vi "FDTI_DX22_read_write.vi"(0 "Handle":u64, 1 "Bytes to wait for":i32, 2 "Read Answer?":bool, 3 "Bytes wait timeout / ms":i32, 5 "Clear  RxTx Buffer?":bool, 7 "Write string":string, 11 "error in (no error)":errorcluster) -> (4 "Handle out":u64, 8 "Read Data":string, 15 "error out":errorcluster)   [LabVIEW 2019]
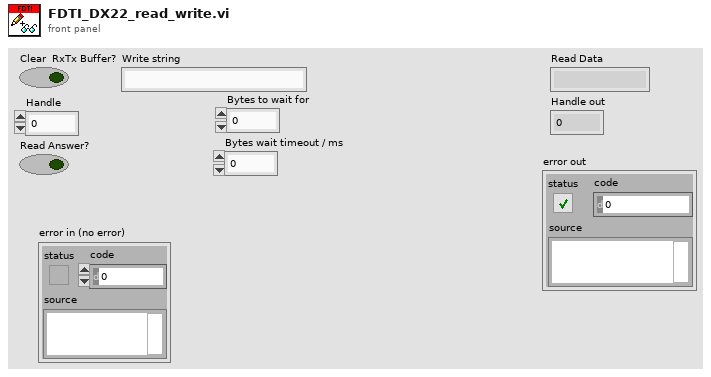
[diagram p1: front panel]
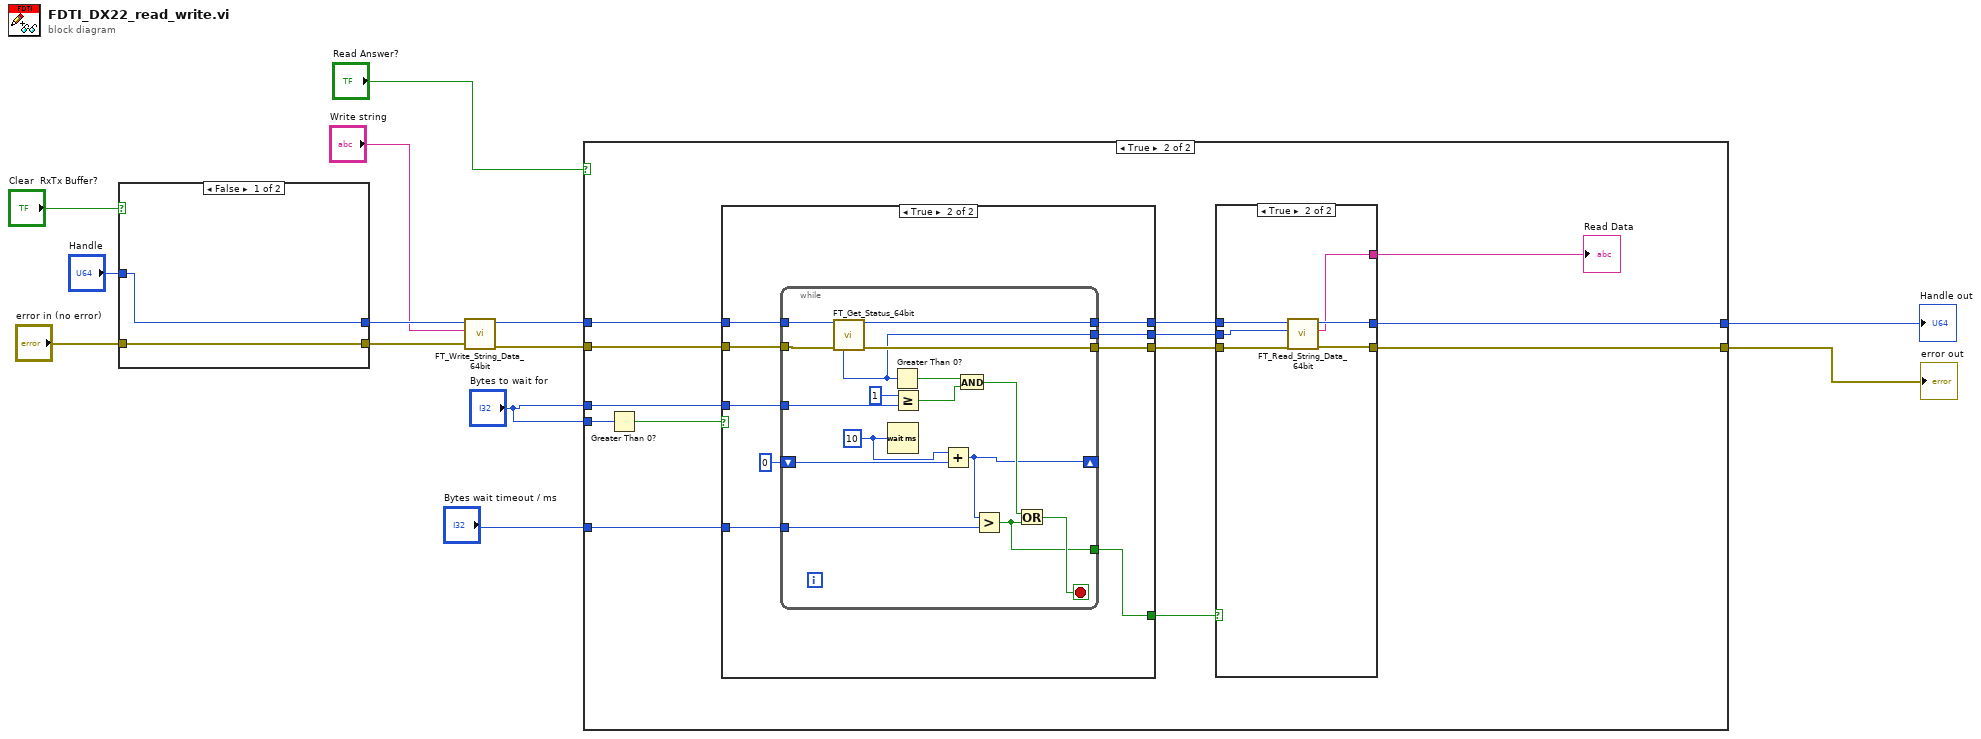
[diagram p0: block diagram]
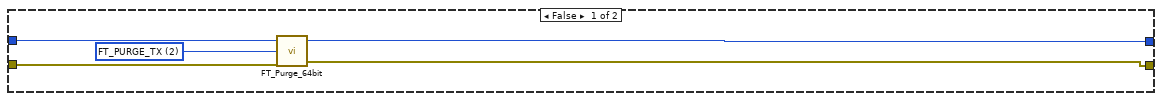
[diagram p2: hidden frame]
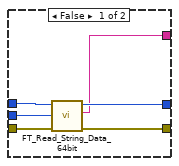
[diagram p3: hidden frame]
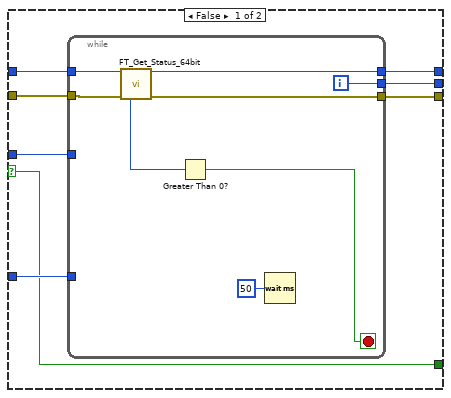
[diagram p4: hidden frame]
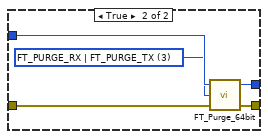
[diagram p5: hidden frame]
diagram:
  n1 = case shown="False" "Clear  RxTx Buffer?" {
    tunnel: "Handle" -> [w15 w20]
    tunnel: [w15 w19] -> w10
    tunnel: "error in (no error)" -> [w14 w17]
    tunnel: [w14 w16] -> w9
    frame False {
    }
    frame True {
      w18 = u32 3 items=["FT_PURGE_RX"=1, "FT_PURGE_TX"=2, "FT_PURGE_RX | FT_PURGE_TX"=3] ("Purge Flags")
      n2 = call "FT_Purge_64bit.vi"("error in (no error)"=w17, "Purge Flags"=w18, "Handle in"=w20) -> ("error out"=w16:errorcluster, "Handle Out"=w19:u64)  [unwired: 1 out]
    }
  }
  n3 = call "FT_Write_String_Data_64bit.vi"("error in (no error)"=w9, "Buffer"="Write string", "Handle"=w10) -> ("error out"=w4:errorcluster, "Handle out"=w5:u64)  [unwired: 1 in, 2 out]
  n4 = case shown="True" "Read Answer?" {
    tunnel: "Bytes to wait for" -> [_ w38]
    tunnel: "Bytes to wait for" -> [_ w36]
    tunnel: w5 -> [w25 w35]
    tunnel: w4 -> [w24 w34]
    tunnel: "Bytes wait timeout / ms" -> [_ w33]
    tunnel: [w23 w29] -> w2
    tunnel: [w21 w28] -> w1
    frame False {
      w22 = u32 2 items=["FT_PURGE_RX"=1, "FT_PURGE_TX"=2, "FT_PURGE_RX | FT_PURGE_TX"=3] ("Purge Flags")
      n5 = call "FT_Purge_64bit.vi"("error in (no error)"=w24, "Purge Flags"=w22, "Handle in"=w25) -> ("error out"=w21:errorcluster, "Handle Out"=w23:u64)  [unwired: 1 out]
    }
    frame True {
      n6 = Greater Than 0?(x=w38) -> (x > 0?=w37:bool)
      n7 = case shown="True" w37 {
        selector: w37 -> [w54 _]
        tunnel: w36 -> [w56 w73]
        tunnel: w35 -> [w58 w75]
        tunnel: w34 -> [w57 w74]
        tunnel: w33 -> [w55 w71]
        tunnel: [w54 w70] -> w32
        tunnel: [w53 w69] -> w31
        tunnel: [w52 w68] -> w30
        tunnel: [w51 w67] -> w27
        frame False {
          n8 = while {
            tunnel: w58 -> [w66]
            tunnel: w57 -> [w65]
            tunnel: w56 -> [_]
            tunnel: w55 -> [_]
            tunnel: [w64] -> w53
            tunnel: [w63] -> w52
            tunnel: [w59] -> w51
            i -> [w59]
            stop <- w61 stop-if-true
            n9 = call "FT_Get_Status_64bit.vi"("Handle"=w66, "error in (no error)"=w65) -> ("Handle out"=w64:u64, "RX Bytes"=w62:u32, "error out"=w63:errorcluster)  [unwired: 8 in, 3 out]
            n10 = Greater Than 0?(x=w62) -> (x > 0?=w61:bool)
            n11 = Wait (ms)(milliseconds to wait=u32 50) -> ()  [unwired: 1 out]
          }
        }
        frame True {
          n12 = while {
            tunnel: w75 -> [w91]
            tunnel: w74 -> [w90]
            tunnel: w73 -> [w87]
            shift-right: [w83] -> _
            shift-left: u32 0 -> [w86]
            tunnel: w71 -> [w82]
            tunnel: [w81] -> w70
            tunnel: [w79] -> w69
            tunnel: [w78] -> w68
            tunnel: [w76] -> w67
            stop <- w85 stop-if-true
            w77 = u32 10 ("milliseconds to wait")
            n13 = call "FT_Get_Status_64bit.vi"("Handle"=w91, "error in (no error)"=w90) -> ("Handle out"=w79:u64, "RX Bytes"=w76:u32, "error out"=w78:errorcluster)  [unwired: 8 in, 3 out]
            n14 = Wait (ms)(milliseconds to wait=w77) -> ()  [unwired: 1 out]
            n15 = Greater Than 0?(x=w76) -> (x > 0?=w89:bool)
            n16 = Greater Or Equal?(x=1, y=w87) -> (x >= y?=w88:bool)
            n17 = Add(x=w77, y=w86) -> (x+y=w83:u32)
            n18 = And(x=w89, y=w88) -> (x .and. y?=w84:bool)
            n19 = Greater?(x=w83, y=w82) -> (0:w81:bool)
            n20 = Or(x=w84, y=w81) -> (x .or. y?=w85:bool)
          }
        }
      }
      n21 = case shown="True" w32 {
        tunnel: w31 -> [w44 w50]
        tunnel: w30 -> [w43 w49]
        tunnel: [w42 w48] -> w29
        tunnel: [w41 w47] -> w28
        tunnel: w27 -> [w40 w45]
        tunnel: [w39 w46] -> w26
        frame False {
          n22 = call "FT_Read_String_Data_64bit.vi"("error in (no error)"=w43, "Bytes To Read"=w40, "Handle"=w44) -> ("error out"=w41:errorcluster, "Read Data"=w39:string, "Handle out"=w42:u64)  [unwired: 1 in, 1 out]
        }
        frame True {
          n23 = call "FT_Read_String_Data_64bit.vi"("error in (no error)"=w49, "Bytes To Read"=w45, "Handle"=w50) -> ("error out"=w47:errorcluster, "Read Data"=w46:string, "Handle out"=w48:u64)  [unwired: 1 in, 1 out]
        }
      }
      "Read Data" <- w26
    }
  }
  "Handle out" <- w2
  "error out" <- w1
